vi "get_data.vi"(8 "error in (no error)":errorcluster, 11 "DataFrame in":refnum<class "DataFrame.lvclass">) -> (0 "error out":errorcluster, 2 "data":string, 3 "DataFrame out":refnum<class "DataFrame.lvclass">)   [LabVIEW 2017, in "DataFrame.lvclass"]
uses:
  DataFrame.lvclass
  DataFrame.lvclass/DataFrame.ctl
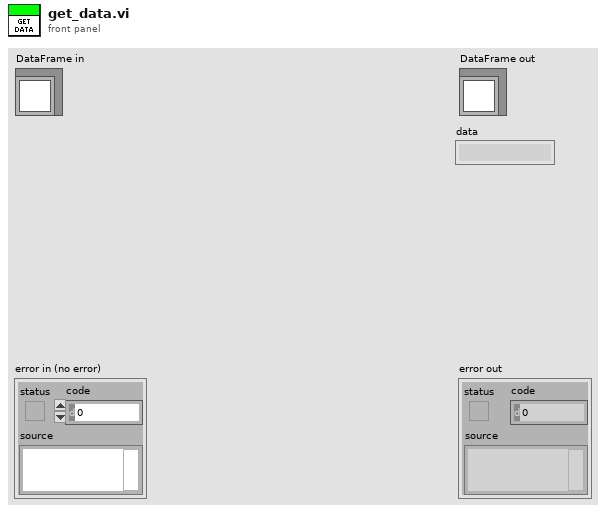
[diagram p1: front panel]
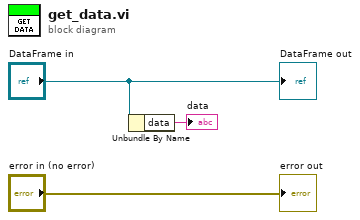
[diagram p0: block diagram]
diagram:
  n1 = Unbundle By Name("DataFrame in") -> ("data"=→"data":string)
  "error out" <- "error in (no error)"
  "DataFrame out" <- "DataFrame in"
